vi "Initial_Auto_Main.vi"() -> ()   [LabVIEW 2017]
uses:
  Destination.ctl
  Start Position.ctl
panel:
  in  "Start Position":T1
  in  "Destination":T2
  # "Initial Autonomous Mode FRC 2018"
  # "This program starts the initial autonomous mode for the FIRST Robotics Competition 2018. The operator selects the start position (A, B, C) and destination (1, 2, 3, 4) from the front panel, and the robot will navigate to the destination and drop off its block."
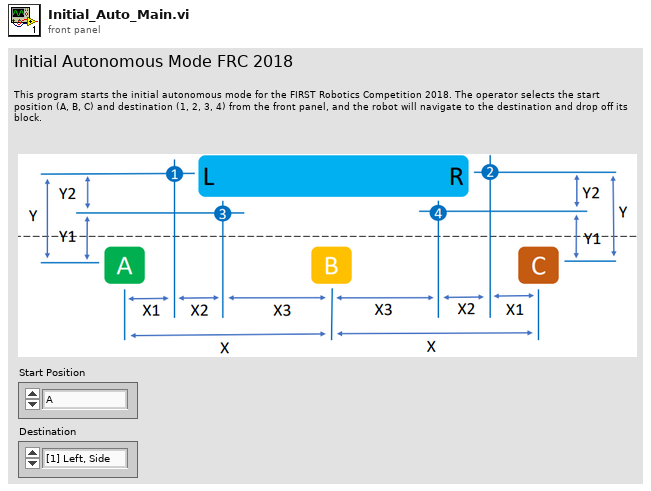
[diagram p1: front panel]
types:
  T1 = typedef "Start Position.ctl" = enum16{"A", "B", "C"}
  T2 = typedef "Destination.ctl" = enum16{"[1] Left, Side ", "[2] Right, Side", "[3] Left, Front", "[4] Right, Front"}
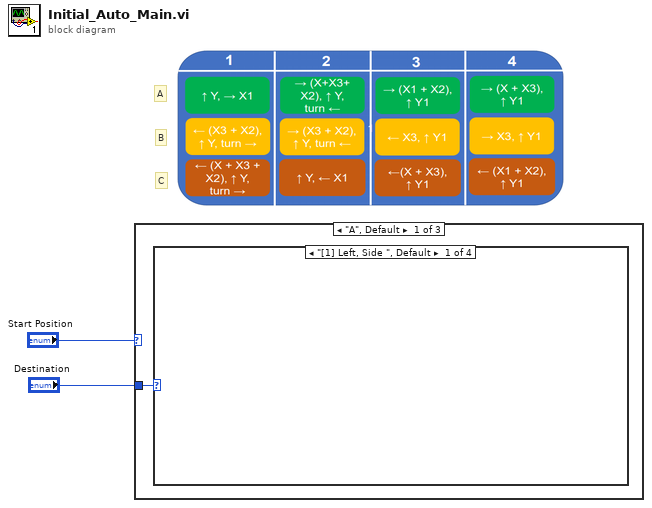
[diagram p0: block diagram]
diagram:
  # "C"
  # "B"
  # "A"
  n1 = case shown="\"A\", Default" "Start Position" {
    tunnel: "Destination" -> [w3 w4 w5]
    frame "A", Default {
      n2 = case shown="\"[1] Left, Side \", Default" w3 {
        frame "[1] Left, Side ", Default {
        }
        frame "[2] Right, Side" {
        }
        frame "[3] Left, Front" {
        }
        frame "[4] Right, Front" {
        }
      }
    }
    frame "B" {
      n3 = case shown="\"[1] Left, Side \", Default" w4 {
        frame "[1] Left, Side ", Default {
        }
        frame "[2] Right, Side" {
        }
        frame "[3] Left, Front" {
        }
        frame "[4] Right, Front" {
        }
      }
    }
    frame "C" {
      n4 = case shown="\"[1] Left, Side \", Default" w5 {
        frame "[1] Left, Side ", Default {
        }
        frame "[2] Right, Side" {
        }
        frame "[3] Left, Front" {
        }
        frame "[4] Right, Front" {
        }
      }
    }
  }
